vi "State History.vi"(7 "history length (100)":i32=100, 11 "Current State":string) -> (3 "History":string)   [LabVIEW 2019]
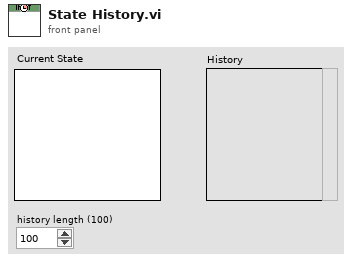
[diagram p1: front panel]
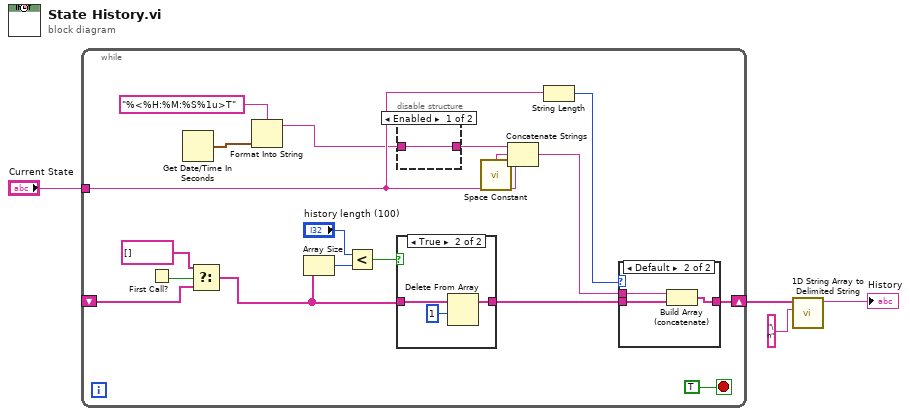
[diagram p0: block diagram]
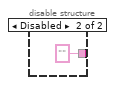
[diagram p2: hidden frame]
diagram:
  n1 = while {
    tunnel: "Current State" -> [w18]
    shift-right: [w19] -> w2
    shift-left: _ -> [w7]
    stop <- TRUE stop-if-true
    n2 = First Call?() -> (First Call?: T/F=w8:bool)
    n3 = Get Date/Time In Seconds() -> (seconds since 1Jan1904=w11:timestamp)
    n4 = Select(t=string[] [], s=w8, f=w7) -> (s? t:f=w6:string[])
    n5 = Format Into String(format string="%<%H:%M:%S%1u>T", w11) -> (resulting string=w9:string)  [unwired: 2 in, 1 out]
    n6 = Array Size(array=w6) -> (size(s)=w21:i32)
    n7 = Less?(x="history length (100)", y=w21) -> (x < y?=w15:bool)
    n8 = case shown="True" w15 {
      tunnel: w6 -> [w29 w30]
      tunnel: [w29 w31] -> w22
      frame False {
      }
      frame True {
        n9 = Delete From Array(array=w30, length=1) -> (array with subset deleted=w31:string[])  [unwired: 1 in, 1 out]
      }
    }
    n10 = disable-structure shown="Enabled" {
      disable-tunnel: [w23 "" ("Spinner Out")] -> w17
      disable-tunnel: w9 -> [w23 _]
      frame Enabled {
      }
      frame Disabled {
      }
    }
    n11 = call <vilib>:"Space Constant.vi"() -> ("String"=w16:string)
    n12 = Concatenate Strings(w17, w16, w18) -> (w14:string)
    n13 = String Length(string=w18) -> (length=w13:i32)
    n14 = case shown="Default" w13 {
      tunnel: w22 -> [w25 w27]
      tunnel: [w25 w28] -> w19
      tunnel: w14 -> [_ w26]
      frame 0 {
      }
      frame Default {
        n15 = Build Array (concatenate)(w26, w27) -> (w28:string[])
      }
    }
  }
  n16 = call <vilib>:"1D String Array to Delimited String.vi"("delimiter"="\n", "string array"=w2) -> ("delimited string"=→"History":string)  [unwired: 9 in]
